vi "Flat Field Correction.vi"() -> ()   [LabVIEW 2016]
uses:
  <vilib>/vision/NI_Vision_Development_Module.lvlib
panel:
  in  "Tab":enum32{"Src", "Flat Field", "Correcte"}(tab)
  out "Src":T1(plugin-control)
  out "FlatField":T1(plugin-control)
  out "Corrected":T1(plugin-control)
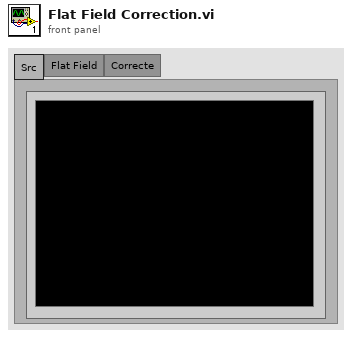
[diagram p1: front panel]
types:
  T1 = typedef "IMAQ Image.ctl" = refnum<image>
  T2 = cluster{"Line Scan Image?":bool, "Correction Factor":sgl}
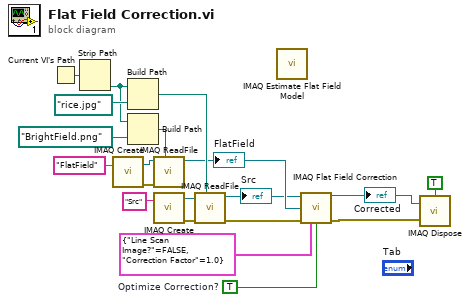
[diagram p0: block diagram]
diagram:
  w5 = TRUE  # Optimize Correction?
  n1 = Current VI's Path() -> (path=w16:path)
  n2 = Strip Path(path=w16) -> (stripped path=w12:path)  [unwired: 1 out]
  n3 = call "IMAQ Create"("Image Name"="FlatField") -> ("New Image"=w8:T1, "error out"=w10:errorcluster)  [unwired: 4 in]
  n4 = Build Path(base path=w12, name or relative path=path "rice.jpg" ("prompt")) -> (appended path=w13:path)
  n5 = Build Path(base path=w12, name or relative path=path "BrightField.png" ("prompt")) -> (appended path=w7:path)
  n6 = call "IMAQ ReadFile"("File Path"=w7, "error in (no error)"=w10, "Image"=w8) -> ("Image Out"=w2:T1)  [unwired: 4 in, 4 out]
  "FlatField" <- w2
  n7 = call "IMAQ Create"("Image Name"="Src") -> ("New Image"=w20:T1, "error out"=w19:errorcluster)  [unwired: 4 in]
  n8 = call "IMAQ ReadFile"("File Path"=w13, "error in (no error)"=w19, "Image"=w20) -> ("error out"=w14:errorcluster, "Image Out"=w1:T1)  [unwired: 4 in, 3 out]
  "Src" <- w1
  n9 = call "IMAQ Estimate Flat Field Model"() -> ()  [unwired: 14 in, 2 out]
  n10 = call "IMAQ Flat Field Correction"("Image Src"=w1, "Flat Field Image"=w2, "error in (no error)"=w14, "Correction Options"=T2 {"Line Scan Image?"=FALSE, "Correction Factor"=1.0}, "Optimize Correction?"=w5) -> ("Corrected Image"=w3:T1, "error out"=w4:errorcluster)  [unwired: 8 in, 1 out]
  "Corrected" <- w3
  n11 = call "IMAQ Dispose"("All Images? (No)"=TRUE, "Image"=w3, "error in (no error)"=w4) -> ()  [unwired: 3 in, 1 out]
